vi "Gamma_upd.vi"(3 "error in (no error)":errorcluster, 4 "\\lambda":dbl, 5 "P(t-1)":T1) -> (0 "error out":errorcluster, 2 "Gamma(t)":T1)   [LabVIEW 2021]
uses:
  <vilib>/Analysis/Matrix/Datatypes/RealMatrix.ctl
  <vilib>/Analysis/Matrix/Numeric/Multiply/Multiply - RM,R.vi
  <vilib>/Analysis/Matrix/NI_Matrix.lvlib
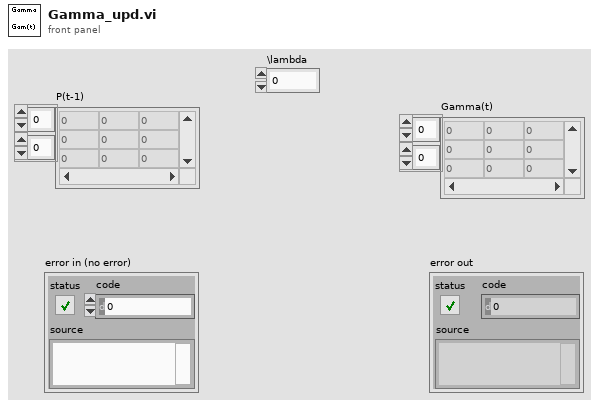
[diagram p1: front panel]
types:
  T1 = typedef "NI_Matrix.lvlib/RealMatrix.ctl" = dbl[][]
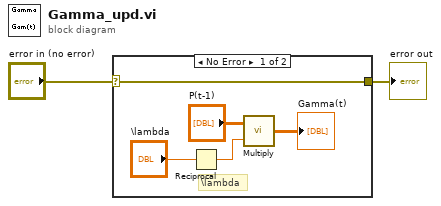
[diagram p0: block diagram]
diagram:
  n1 = case shown="No Error" "error in (no error)" {
    selector: "error in (no error)" -> [w4 w8]
    tunnel: [w4 w8] -> w1
    frame No Error {
      # "\\lambda"
      n2 = Reciprocal(x="\\lambda") -> (1/x=w7:dbl)
      n3 = call-poly <vilib>:"Multiply.vi"("Real Scalar c"=w7, "Real Matrix A"="P(t-1)") -> ("A * c"=→"Gamma(t)":T1)
    }
    frame Error {
    }
  }
  "error out" <- w1
